vi "FGV Semaforo.vi"(10 "semaphore":T1, 11 "Function":enum16{"GET", "SET"}(ring)) -> (2 "semaphore out":T1)   [LabVIEW 2015]
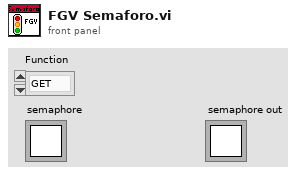
[diagram p1: front panel]
types:
  T1 = typedef "Semaphore RefNum" = refnum<k1>
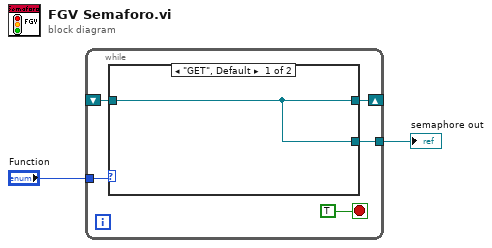
[diagram p0: block diagram]
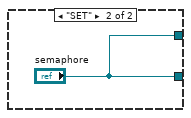
[diagram p2: hidden frame]
diagram:
  n1 = while {
    tunnel: "Function" -> [w6]
    shift-right: [w4] -> _
    shift-left: _ -> [w5]
    tunnel: [w3] -> w1
    stop <- TRUE stop-if-true
    n2 = case shown="\"GET\", Default" w6 {
      tunnel: w5 -> [w8 _]
      tunnel: [w8 "semaphore"] -> w4
      tunnel: [w8 "semaphore"] -> w3
      frame "GET", Default {
      }
      frame "SET" {
      }
    }
  }
  "semaphore out" <- w1
